vi "setPrecision.vi"(9 "Precision":u32, 10 "Number":dbl format="%#.12g") -> (2 "Rounded Number":dbl)   [LabVIEW 2011]
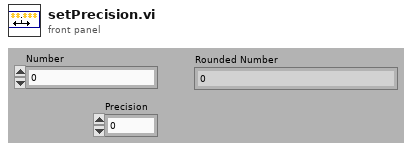
[diagram p1: front panel]
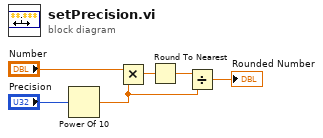
[diagram p0: block diagram]
diagram:
  n1 = Power Of 10(x="Precision") -> (10^x=w2:dbl)
  n2 = Multiply(x="Number", y=w2) -> (x*y=w4:dbl)
  n3 = Round To Nearest(number=w4) -> (nearest integer value=w3:dbl)
  n4 = Divide(x=w3, y=w2) -> (x/y=→"Rounded Number":dbl)
